vi "Call NIPKG CLI (runas admin).vi"(8 "error in (no error)":errorcluster, 11 "command":string) -> (0 "error out":errorcluster)   [LabVIEW 2021, in "NIPM_API.lvlib"]
doc: "This VI calls the nipkg.exe command-line interface (CLI) from the command line as an admin.\n\nNotes:\nThis VI will launch a Windows dialog asking for permission to run and requires the user to have admin rights. This VI uses the ShellExecuteA function in <system32>\\shell32.dll.\n\nThis VI will not return an error if the nipkg command failed. This VI only returns an error if the ShellExecuteA function itself has an error.\n\nINPUT(s)\n<B>Command</B> is a string containing the specific nipkg CLI command (e.g. install, remove) to execute as an admin."
uses:
  NIPM_API.lvlib
  <vilib>/Utility/sysdir.llb/System Directory Type.ctl
panel:
  out "HINSTANCE":i32
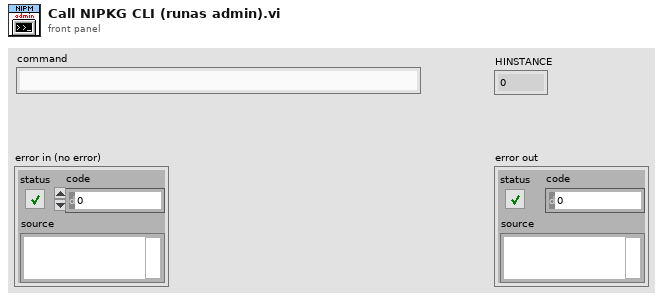
[diagram p1: front panel]
types:
  T1 = typedef "System Directory Type.ctl" = i32
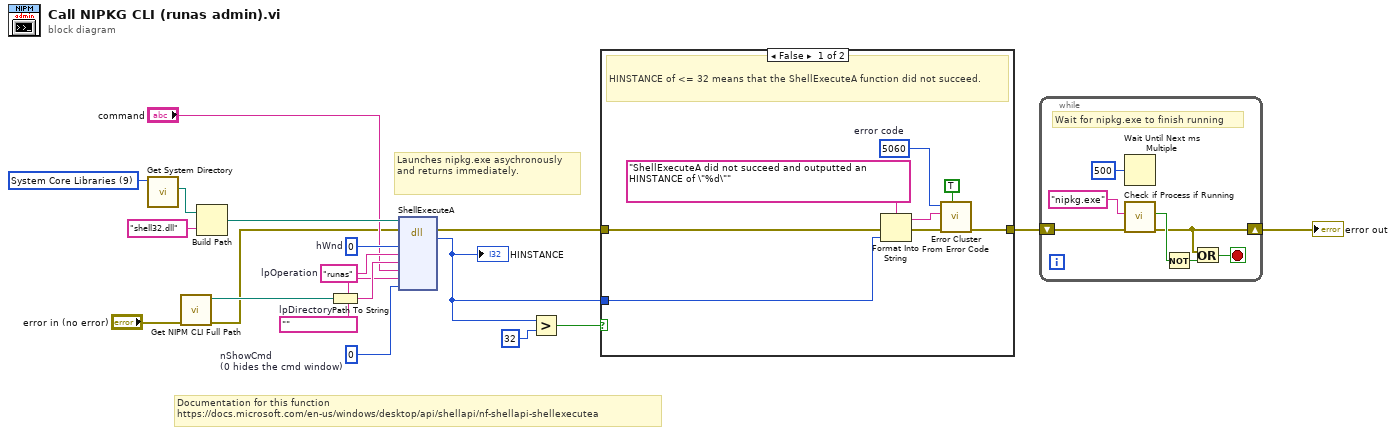
[diagram p0: block diagram]
diagram:
  w10 = 0  # nShowCmd (0 hides the cmd window)
  w11 = ""  # lpDirectory
  w14 = "runas"  # lpOperation
  w15 = 0  # hWnd
  w19 = T1 9 items=["User Home"=0, "User Desktop"=1, "User Documents"=2, "User Application Data"=3, "User Preferences"=4, "User Temporary"=5, "Public Documents"=6, "Public Application Data"=7, "Public Preferences"=8, "Public Cache"=13, "System Core Libraries"=9, "System Installed Libraries"=10, "Application Files"=11, "Boot Volume Root"=12] ("system directory type")
  # "Launches nipkg.exe asychronously and returns immediately."
  # "Documentation for this function\nhttps://docs.microsoft.com/en-us/windows/desktop/api/shellapi/nf-shellapi-shellexecutea"
  n1 = call <vilib>:"Get System Directory.vi"("system directory type"=w19) -> ("system directory"=w18:path)  [unwired: 10 in]
  n2 = call "Get NIPM CLI Full Path.vi"("error in (no error)"="error in (no error)") -> ("error out"=w1:errorcluster, "NIPM CLI"=w3:path)  [unwired: 9 in]
  n3 = Build Path(base path=w18, name or relative path="shell32.dll") -> (appended path=w16:path)
  n4 = Path To String(path=w3) -> (string=w13:string)
  n5 = dll-call lib="C:/Windows/System32/shell32.dll" fn="ShellExecuteA"(path in=w16, error in=w1, "hWnd"=w15, "lpOperation"=w14, "lpFile"=w13, "lpParameters"="command", "lpDirectory"=w11, "nShowCmd"=w10) -> (error out=w7:errorcluster, "HINSTANCE"=w6:i32)  [unwired: 7 in, 1 out]
  "HINSTANCE" <- w6
  n6 = Greater?(x=w6, y=32) -> (0:w8:bool)
  n7 = case shown="False" w8 {
    tunnel: w7 -> [w22 w28]
    tunnel: [w25 w28] -> w5
    tunnel: w6 -> [w23 _]
    frame False {
      w26 = 5060  # error code
      # "HINSTANCE of <= 32 means that the ShellExecuteA function did not succeed."
      n8 = Format Into String(format string="ShellExecuteA did not succeed and outputted an HINSTANCE of \"%d\"" ("error message (\"\")"), error in=w22, w23) -> (resulting string=w20:string, error out=w21:errorcluster)  [unwired: 1 in]
      n9 = call <vilib>:"Error Cluster From Error Code.vi"("show call chain? (False)"=TRUE, "error in (no error)"=w21, "error message (\"\")"=w20, "error code (0)"=w26) -> ("error out"=w25:errorcluster)  [unwired: 5 in]
    }
    frame True {
      # "ShellExecuteA did not return an error"
    }
  }
  n10 = while {
    shift-right: [w30] -> w4
    shift-left: w5 -> [w34]
    stop <- w29 stop-if-true
    # "Wait for nipkg.exe to finish running"
    # "Wait for nipkg.exe to finish running"
    n11 = Wait Until Next ms Multiple(millisecond multiple=u32 500) -> ()  [unwired: 1 out]
    n12 = call "Check if Process if Running.vi"("error in (no error)"=w34, "Process Name"="nipkg.exe") -> ("error out"=w30:errorcluster, "Running?"=w33:bool)  [unwired: 8 in]
    n13 = Not(x=w33) -> (.not. x?=w31:bool)
    n14 = Or(x=w30, y=w31) -> (x .or. y?=w29:bool)
  }
  "error out" <- w4
